vi "Y data to Force extension.vi"() -> ()   [LabVIEW 2012]
panel:
  out "Fit Results":T1
  in  "DNA length (µm)":dbl=0.658
  in  "fsampling (Hz)":dbl=2800.0
  in  "X/Y data":dbl[](array[numeric])
  in  "Fit settings":T2={"#PSD Averages"=40, "Correct camera acquisition artifacts"=TRUE, "Autorange"=TRUE, "fstart (Hz)"=0.0, "Pendulum geometry"=FALSE, "Fit model"=FALSE} {"#PSD Averages" min=1}
  # "Fit parameters"
  # "Calculated quantities"
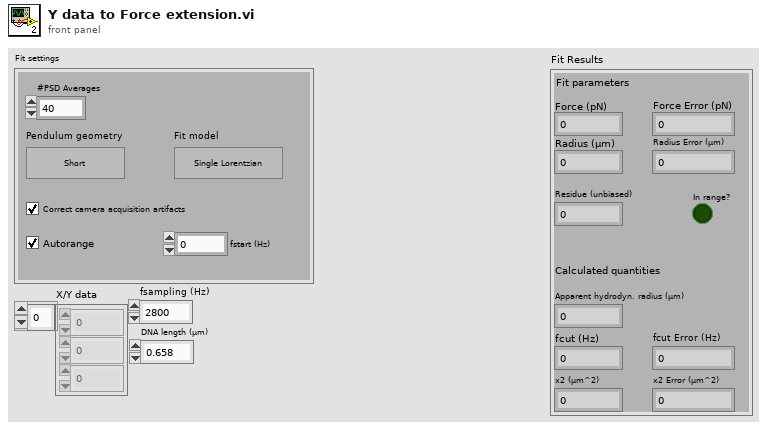
[diagram p1: front panel]
types:
  T1 = cluster{"fcut (Hz)":dbl, "x2 (µm^2)":dbl, "Force (pN)":dbl, "Radius (µm)":dbl, "Apparent hydrodyn. radius (µm)":dbl, "fcut Error (Hz)":dbl, "x2 Error (µm^2)":dbl, "Force Error (pN)":dbl, "Radius Error (µm)":dbl, "Residue (unbiased)":dbl, "In range?":bool}
  T2 = cluster{"#PSD Averages":u8, "Correct camera acquisition artifacts":bool, "Autorange":bool, "fstart (Hz)":dbl, "Pendulum geometry":bool, "Fit model":bool}
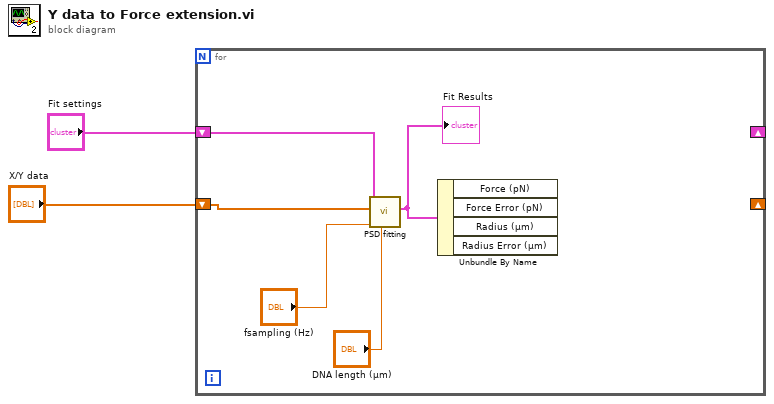
[diagram p0: block diagram]
diagram:
  n1 = for {
    shift-right: _ -> [_]
    shift-left: "Fit settings" -> [w7]
    shift-right: _ -> [_]
    shift-left: "X/Y data" -> [w3]
    n2 = call "PSD fitting.vi"("DNA length (µm)"="DNA length (µm)", "fsampling (Hz)"="fsampling (Hz)", "Fit settings"=w7, "X/Y data"=w3) -> ("Fit Results"=w6:T1)  [unwired: 7 in]
    "Fit Results" <- w6
    n3 = Unbundle By Name(w6) -> ()  [unwired: 4 out]
  }
